vi "Get_Vi_Data_loop.vi"(8 "Data Type":u16(ring) items=["String", "Double", "Boolean", "Variant"], 9 "vi reference in":refnum<vi>, 10 "Control Name":string, 11 "application reference in":refnum<vi>) -> (0 "application reference out":refnum<vi>, 1 "Boolean":bool, 2 "Data (Double)":dbl format="%#_4g", 3 "Data (String)":string, 4 "vi reference out":refnum<vi>, 5 "Data (Variant)":variant, 6 "error out":errorcluster)   [LabVIEW 2021]
panel:
  in  "error in (no error)":errorcluster
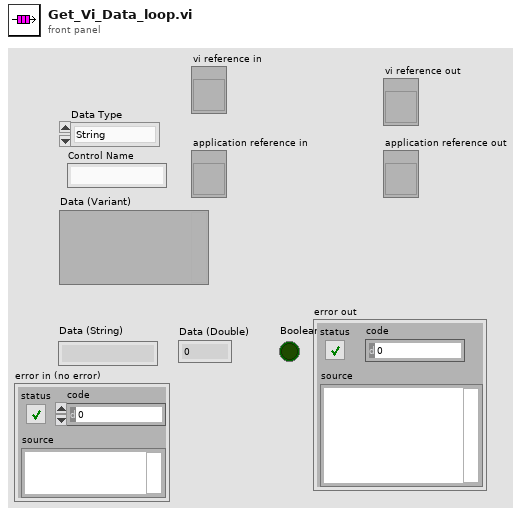
[diagram p1: front panel]
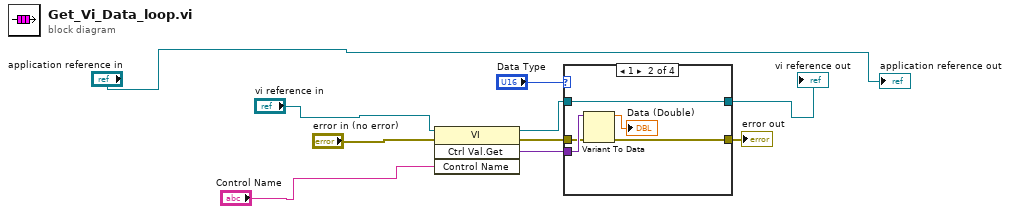
[diagram p0: block diagram]
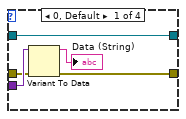
[diagram p2: hidden frame]
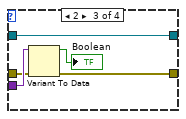
[diagram p3: hidden frame]
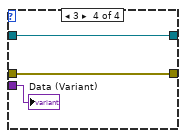
[diagram p4: hidden frame]
diagram:
  n1 = invoke class="VI" method="Ctrl Val.Get"(reference="vi reference in", error in="error in (no error)", "Control Name"="Control Name") -> (reference out=w4:refnum<vi>, error out=w5:errorcluster, "Get Control Value Variant"=w6:variant)  [unwired: 1 in, 1 out]
  n2 = case shown="1" "Data Type" {
    tunnel: w6 -> [w15 w20 w25 w28]
    tunnel: w5 -> [w14 w19 w24 w27]
    tunnel: w4 -> [w11 w16 w21 w26]
    tunnel: [w12 w17 w22 w27] -> w1
    tunnel: [w11 w16 w21 w26] -> w9
    frame 0, Default {
      n3 = Variant To Data(error in=w14, Variant=w15) -> (data=→"Data (String)":string, error out=w12:errorcluster)  [unwired: 1 in]
    }
    frame 1 {
      n4 = Variant To Data(error in=w19, Variant=w20) -> (data=→"Data (Double)":dbl, error out=w17:errorcluster)  [unwired: 1 in]
    }
    frame 2 {
      n5 = Variant To Data(error in=w24, Variant=w25) -> (data=→"Boolean":bool, error out=w22:errorcluster)  [unwired: 1 in]
    }
    frame 3 {
      "Data (Variant)" <- w28
    }
  }
  "vi reference out" <- w9
  "error out" <- w1
  "application reference out" <- "application reference in"
